vi "PH_Cont-601k_PSU.Dev Set Configuration.vi"(0 "VI in":refnum<vi>, 5 "error in (no error)":errorcluster) -> (14 "VI out":refnum<vi>, 18 "Device Error out":errorcluster, 19 "error out":errorcluster)   [LabVIEW 2014, in "PH_Cont-601k_PSU.lvlib"]
uses:
  PH_Cont-601k_PSU.lvlib
  instr.lib/pu601k/Continuum PU610K.lvlib
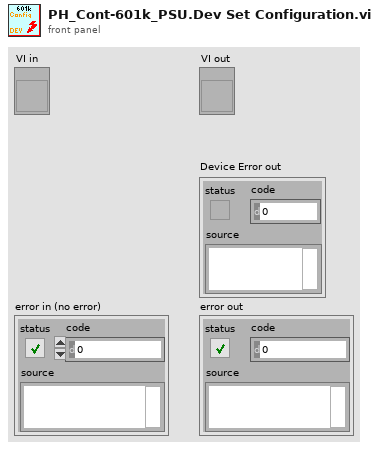
[diagram p1: front panel]
types:
  T1 = typedef "PH_Cont-601k_PSU.lvlib/PH_Cont-601k_PSU.i attribute.ctl" = cluster{"GUI Refs":T2, "Interlock":bool, "Service ID applied Voltage":i32, "Device Settings":cluster{"Configuration":T3, "Flash Interval [s]":dbl, "Mode":T4, "Voltage [V]":u16, "Charge":bool, "VISA resource name":refnum<visa-resource-name>}, "Readyness":T5, "Information":cluster{"VISA resource name":refnum<visa-resource-name>, "Tagname Power On":string, "Interlock":cluster{"Instance":string, "Tagname":string}, "Limits [V]":cluster{"Lower":dbl, "Upper":dbl}, "Tagname PSU On":string}, "R2S":bool, "Charge is allowed":bool}
  T2 = typedef "PH_Cont-601k_PSU.lvlib/PH_Cont-601k_PSU.GUI Refs.ctl" = cluster{"Power On":refnum<vi>, "Hard- and Software":refnum<vi>, "Device Status":refnum<vi>, "Device Error":refnum<vi>, "Configuration":refnum<vi>, "Flash Interval [s]":refnum<vi>, "Interlock":refnum<vi>, "Interlock Indicator":refnum<vi>, "Voltage [V]":refnum<vi>, "Readyness":refnum<vi>, "Mode":refnum<vi>, "Reset Error":refnum<vi>, "Expert working":refnum<vi>, "Charge":refnum<vi>, "PSU On":refnum<vi>}
  T3 = typedef "PH_Cont-601k_PSU.lvlib/PH_Cont-601k_PSU.Configuration.ctl" = u16
  T4 = typedef "PH_Cont-601k_PSU.lvlib/PH_Cont-601k_PSU.Mode.ctl" = enum32{"STOP", "STANDBY", "READY", "EMISSION", "ERROR"}
  T5 = typedef "PH_Cont-601k_PSU.lvlib/PH_Cont-601k_PSU.Readyness.ctl" = cluster{"Program":T6, "Device":T7}
  T6 = typedef "PH_Cont-601k_PSU.lvlib/PH_Cont-601k_PSU.Readyness Program.ctl" = enum32{"OFF", "POWER", "INTERLOCK"}
  T7 = typedef "PH_Cont-601k_PSU.lvlib/PH_Cont-601k_PSU.Readyness Device.ctl" = enum32{"OFF", "CONNECTING", "CONNECTED", "OPERATING", "EOC", "ERROR"}
  T8 = enum16{"Ch intl, Fl intl, QSw intl", "Ch intl, Fl intl, QSw ext", "Ch intl, Fl ext, QSw intl", "Ch intl, Fl ext, QSw ext", "Ch ext, Fl int, QSw int", "Ch ext, Fl int, QSw ext", "Ch ext, Fl ext, QSw int", "Ch ext, Fl ext, QSw ext"}
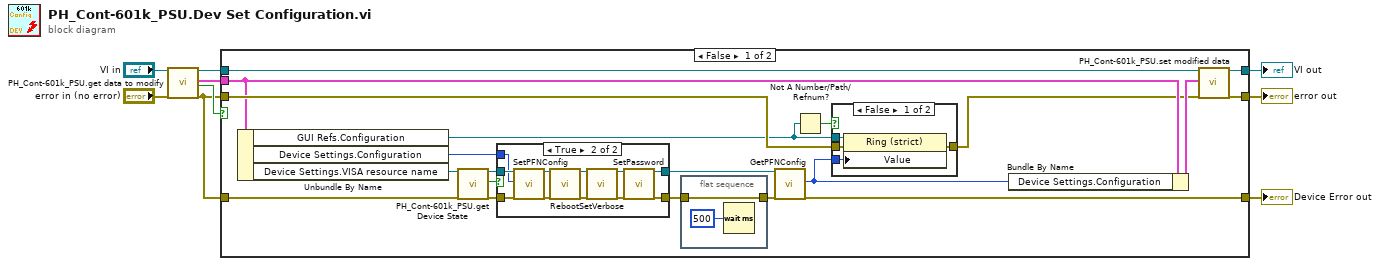
[diagram p0: block diagram]
diagram:
  n1 = call "PH_Cont-601k_PSU.get data to modify.vi"("i ref in"="VI in", "error in (no error)"="error in (no error)") -> ("i ref out"=w5:refnum<vi>, "i attribute"=w8:T1, "timed out"=w2:bool, "error out"=w1:errorcluster)  [unwired: 14 in]
  n2 = case shown="False" w2 {
    tunnel: [w16 w50] -> w9
    tunnel: w1 -> [w26 w50]
    tunnel: w8 -> [w21 _]
    tunnel: w5 -> [w25 w52]
    tunnel: [w24 w52] -> w4
    tunnel: w1 -> [w23 w51]
    tunnel: [w22 w51] -> w3
    frame False {
      n3 = Unbundle By Name(w21) -> ("GUI Refs.Configuration"=w10:refnum<vi>, "Device Settings.Configuration"=w17:T3, "Device Settings.VISA resource name"=w18:refnum<visa-resource-name>)
      n4 = call "PH_Cont-601k_PSU.get Device State.vi"("VISA Refnum in"=w18, "Device Error in"=w26) -> ("VISA Refnum out"=w29:refnum<visa-resource-name>, "Configuration Change is allowed"=w27:bool, "Device Error out"=w28:errorcluster)  [unwired: 9 in, 6 out]
      n5 = case shown="True" w27 {
        tunnel: [w38 w41] -> w19
        tunnel: w29 -> [w37 w43]
        tunnel: w28 -> [w38 w42]
        tunnel: w17 -> [_ w40]
        tunnel: [w37 w39] -> w14
        frame False {
        }
        frame True {
          n6 = call "SetPFNConfig.vi"("VISA resource name"=w43, "PFN Mode"=w40, "error in"=w42) -> ("VISA resource name out"=w44:refnum<visa-resource-name>, "error out"=w45:errorcluster)  [unwired: 15 in]
          n7 = call "Reboot.vi"("VISA resource name"=w44, "error in"=w45) -> ("VISA resource name out"=w46:refnum<visa-resource-name>, "error out"=w48:errorcluster)  [unwired: 16 in]
          n8 = call "SetVerbose.vi"("VISA resource name"=w46, "error in"=w48) -> ("VISA resource name out"=w47:refnum<visa-resource-name>, "error out"=w49:errorcluster)  [unwired: 16 in]
          n9 = call "SetPassword.vi"("VISA resource name"=w47, "error in"=w49) -> ("VISA resource name out"=w39:refnum<visa-resource-name>, "error out"=w41:errorcluster)  [unwired: 16 in]
        }
      }
      n10 = flat-sequence {
        tunnel: w19 -> [w36]
        tunnel: [w36] -> w15
        frame #0 {
          n11 = Wait (ms)(milliseconds to wait=u32 500) -> ()  [unwired: 1 out]
        }
      }
      n12 = call "GetPFNConfig.vi"("VISA resource name"=w14, "error in"=w15) -> ("PFN Mode"=w12:T8, "error out"=w16:errorcluster)  [unwired: 15 in, 1 out]
      n13 = Not A Number/Path/Refnum?(number/path/refnum=w10) -> (NaN/Path/Refnum?=w11:bool)
      n14 = case shown="False" w11 {
        tunnel: w23 -> [w33 w34]
        tunnel: [w32 w34] -> w13
        tunnel: w10 -> [w31 _]
        tunnel: w12 -> [w30 _]
        frame False {
          n15 = property class="Ring (strict)"(reference=w31, error in=w33, "Value"=w30) -> (error out=w32:errorcluster)  [unwired: 1 out]
        }
        frame True {
        }
      }
      n16 = Bundle By Name(cluster=w21, "Device Settings.Configuration"=w12) -> (w20:T1)
      n17 = call "PH_Cont-601k_PSU.set modified data.vi"("i ref in"=w25, "i attribute"=w20, "error in (no error)"=w13) -> ("i ref out"=w24:refnum<vi>, "error out"=w22:errorcluster)  [unwired: 15 in]
    }
    frame True {
    }
  }
  "error out" <- w3
  "VI out" <- w4
  "Device Error out" <- w9
